vi "Initialize Generate.vi"(8 "error in (no error)":errorcluster, 10 "PCL (usec)":u32, 11 "OnCompile Variables":T12={"Name"="", "XNET Settings"={"Database"="", "Cluster"="", "Port"="", "Baud rate [Bd]"=500000, "Termination"=1, "CAN I/O Mode"=0, "FD Baud rate [Bd]"=500000, "Priority"=100, "Use Legacy"=FALSE, "FD ISO Mode"=0}, "Frames"=[], "986x Support"={"Enable"=FALSE, "RIO Device"="", "Bitfile"=path ""}, "Incoming Signal Info"={"Signal Settings Out"=[], "Signal_Valid_Values"=[], "Signal Names"=[]}, "Incoming Frames"=[]} {"Incoming Frames"."Protection Configurations"."CRC Channels"."Data Type" items=["Signed", "Unsigned", "IEEE Float"]; "Incoming Signal Info"."Signal Settings Out"."Protection Configuration"."CRC Channels"."Data Type" items=["Signed", "Unsigned", "IEEE Float"]; "XNET Settings"."FD ISO Mode" items=["ISO", "Non ISO", "ISO Legacy"]; "XNET Settings"."CAN I/O Mode" items=["CAN 2.0", "CAN FD", "CAN FD+BRS"]; "XNET Settings"."Termination" items=["Off", "On"]; "Frames"."Protection Configurations"."CRC Channels"."Data Type" items=["Signed", "Unsigned", "IEEE Float"]}) -> (0 "error out":errorcluster, 3 "RT Configuration":T1={"Name"="", "Priority"=100, "CAN Session"="", "Frame Count"=0, "Frames"=[], "FPGA Session"=0, "XNET Settings"={"Database"="", "Cluster"="", "Port"="", "Baud rate [Bd]"=0, "Termination"=0, "CAN I/O Mode"=0, "FD Baud rate [Bd]"=500000, "Priority"=100, "Use Legacy"=FALSE, "FD ISO Mode"=0}, "Incoming Frame Session"="", "Incoming Session Invalid"=FALSE, "Incoming Signal Info"={"Signal_Valid_Values"=[], "Signal Names"=[], "Signal Settings Out"=[], "Frame Receive Time Values"=[]}, "Signal Values"=[]} {"Incoming Signal Info"."Signal Settings Out"."Protection Configuration"."CRC Channels"."Data Type" items=["Signed", "Unsigned", "IEEE Float"]; "XNET Settings"."FD ISO Mode" items=["ISO", "Non ISO", "ISO Legacy"]; "XNET Settings"."CAN I/O Mode" items=["CAN 2.0", "CAN FD", "CAN FD+BRS"]; "XNET Settings"."Termination" items=["Off", "On"]; "Frames"."Protection Configurations"."CRC Channels"."Data Type" items=["Signed", "Unsigned", "IEEE Float"]})   [LabVIEW 2019, in "Protection and Counter Addon Engine.lvlib"]
uses:
  Protection and Counter Addon Engine.lvlib
  Addon Shared/Types/Exported.OnCompile.ctl
  Addon Shared/Types/XNET Settings.ctl
  SubModules/Frame-Protection-Support/Source/Shared/Types/Exported Frame Settings.ctl
  SubModules/Frame-Protection-Support/Source/Shared/Types/Exported Frame Type.ctl
  SubModules/Frame-Protection-Support/Source/Shared/Types/Exported Protection Settings.ctl
  SubModules/Frame-Protection-Support/Source/Shared/Types/Protection Type.ctl
  SubModules/Frame-Protection-Support/Source/Shared/Types/XNET Signal Configuration.ctl
  SubModules/Frame-Protection-Support/Source/Shared/Types/Exported Counter Settings.ctl
  SubModules/Frame-Protection-Support/Source/Shared/Types/Exported Event Trigger Type.ctl
  Addon Shared/Types/986x.ctl
  SubModules/Frame-Protection-Support/Source/Shared/Types/Incoming Signal Info.ctl
  SubModules/Frame-Protection-Support/Source/Shared/Types/Exported Signal Settings.ctl
  Types/RT Async Engine Settings.ctl
  SubModules/Frame-Protection-Support/Source/Engine/Types/RT Frame Settings.ctl
  SubModules/Frame-Protection-Support/Source/Engine/Types/RT Protection Configuration.ctl
  SubModules/Frame-Protection-Support/Source/Shared/Types/RT_Incoming_Signal_Info.ctl
  SubModules/Frame-Protection-Support/Source/Shared/Types/RT Exported Signal Settings.ctl
  <vilib>/xnet/xnet.llb/XNET Create Session (Frame Output Stream).vi
  SubModules/Frame-Protection-Support/Source/Shared/Protection and Counter Support Shared.lvlib
  SubModules/Frame-Protection-Support/Source/Engine/Protection and Counter Support Engine.lvlib
  <resource>/objmgr/xnet.rc
  Addon Shared/Protection and Counter Addon Shared.lvlib
  <vilib>/NI VeriStand/Custom Device Tools/Custom Device Utility Library/Custom Device Utility Library.lvlib
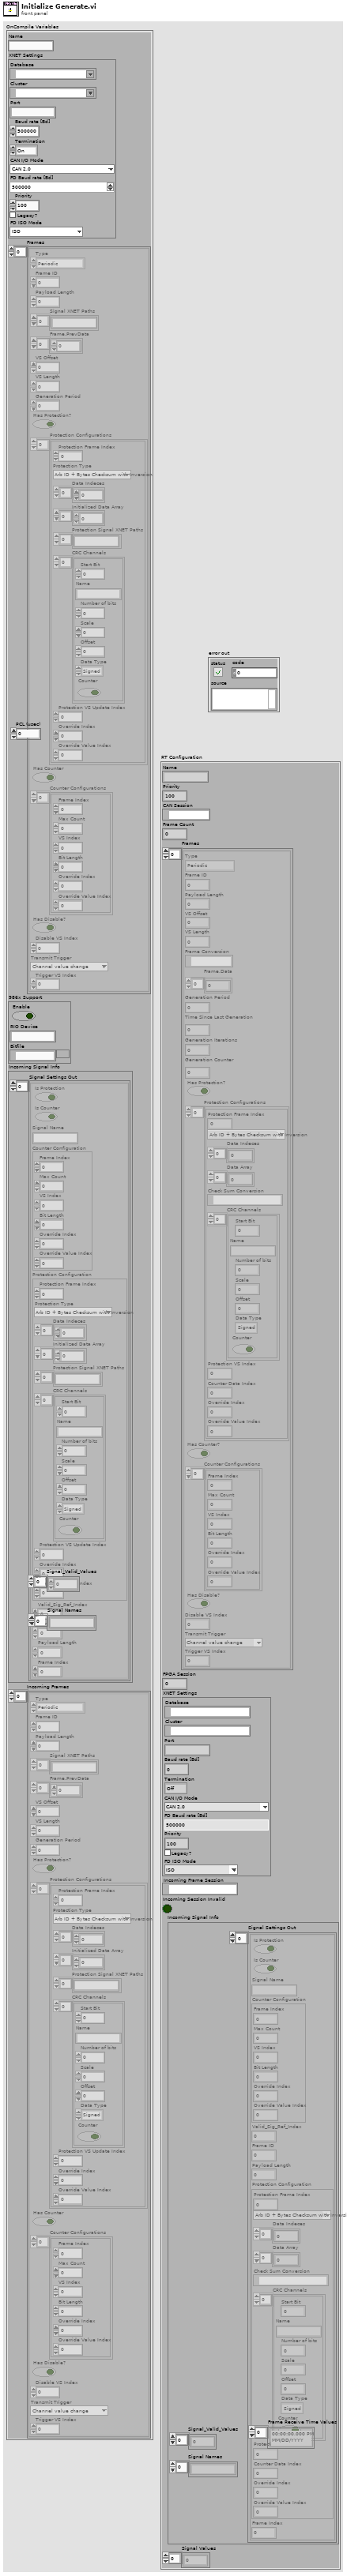
[diagram p1: front panel]
types:
  T1 = typedef "Protection and Counter Addon Engine.lvlib/RT Async Engine Settings.ctl" = cluster{"Name":string, "Priority":i32, "CAN Session":refnum<k21>, "Frame Count":i32, "Frames":T2[], "FPGA Session":u32, "XNET Settings":T9, "Incoming Frame Session":refnum<k21>, "Incoming Session Invalid":bool, "Incoming Signal Info":T10, "Signal Values":dbl[]}
  T2 = typedef "Protection and Counter Support Engine.lvlib/RT Frame Settings.ctl" = cluster{"Type":T3, "Frame ID":u32, "Payload Length":u32, "VS Offset":i32, "VS Length":i32, "Frame Conversion":refnum<k21>, "Frame.Data":dbl[], "Generation Period":u32, "Time Since Last Generation":u32, "Generation Iterations":u32, "Generation Counter":u32, "Has Protection?":bool, "Protection Configurations":T4[], "Has Counter?":bool, "Counter Configurations":T7[], "Has Disable?":bool, "Disable VS Index":i32, "Transmit Trigger":T8, "Trigger VS Index":i32}
  T3 = typedef "Protection and Counter Support Shared.lvlib/Exported Frame Type.ctl" = enum16{"Periodic", "Event", "Periodic/Event"}
  T4 = typedef "Protection and Counter Support Engine.lvlib/RT Protection Configuration.ctl" = cluster{"Protection Frame Index":i32, "Protection Type":T5, "Data Indeces":i32[], "Data Array":dbl[], "Check Sum Conversion":refnum<k21>, "CRC Channels":T6[], "Protection VS Index":i32, "Counter Data Index":i32, "Override Index":i32, "Override Value Index":i32}
  T5 = typedef "Protection and Counter Support Shared.lvlib/Protection Type.ctl" = enum16{"Arb ID + Bytes Checksum with Inversion", "Arb ID + Bytes CRC with Inversion", "Reversed Raw Signal Checksum with Inversion", "Concatenated Two's Compliment"}
  T6 = typedef "Protection and Counter Support Shared.lvlib/XNET Signal Configuration.ctl" = cluster{"Start Bit":i32, "Name":string, "Number of bits":i32, "Scale":dbl, "Offset":dbl, "Data Type":u32, "Counter":bool}
  T7 = typedef "Protection and Counter Support Shared.lvlib/Exported Counter Settings.ctl" = cluster{"Frame Index":i32, "Max Count":dbl, "VS Index":i32, "Bit Length":i64, "Override Index":i32, "Override Value Index":i32}
  T8 = typedef "Protection and Counter Support Shared.lvlib/Exported Event Trigger Type.ctl" = enum16{"Channel value change", "Trigger channel (not zero)", "Channel value change or trigger channel (not zero)", "Trigger channel (any value change)", "Channel value change or trigger channel (any value change)"}
  T9 = typedef "Protection and Counter Addon Shared.lvlib/XNET Settings.ctl" = cluster{"Database":refnum<k21>, "Cluster":refnum<k21>, "Port":string, "Baud rate [Bd]":u64, "Termination":u32, "CAN I/O Mode":u32, "FD Baud rate [Bd]":u64, "Priority":i32, "Use Legacy":bool, "FD ISO Mode":u32}
  T10 = typedef "RT_Incoming_Signal_Info.ctl" = cluster{"Signal_Valid_Values":dbl[], "Signal Names":string[], "Signal Settings Out":T11[], "Frame Receive Time Values":timestamp[]}
  T11 = typedef "RT Exported Signal Settings.ctl" = cluster{"Is Protection":bool, "Is Counter":bool, "Signal Name":string, "Counter Configuration":T7, "Valid_Sig_Ref_Index":i32, "Frame ID":u32, "Payload Length":u32, "Protection Configuration":T4, "Frame Index":i32}
  T12 = typedef "Protection and Counter Addon Shared.lvlib/Exported.OnCompile.ctl" = cluster{"Name":string, "XNET Settings":T9, "Frames":T13[], "986x Support":T15, "Incoming Signal Info":T16, "Incoming Frames":T13[]}
  T13 = typedef "Protection and Counter Support Shared.lvlib/Exported Frame Settings.ctl" = cluster{"Type":T3, "Frame ID":u32, "Payload Length":u32, "Signal XNET Paths":string[], "Frame.PrevData":dbl[], "VS Offset":i32, "VS Length":i32, "Generation Period":u32, "Has Protection?":bool, "Protection Configurations":T14[], "Has Counter":bool, "Counter Configurations":T7[], "Has Disable?":bool, "Disable VS Index":i32, "Transmit Trigger":T8, "Trigger VS Index":i32}
  T14 = typedef "Protection and Counter Support Shared.lvlib/Exported Protection Settings.ctl" = cluster{"Protection Frame Index":i32, "Protection Type":T5, "Data Indeces":i32[], "Initialized Data Array":dbl[], "Protection Signal XNET Paths":string[], "CRC Channels":T6[], "Protection VS Update Index":i32, "Override Index":i32, "Override Value Index":i32}
  T15 = typedef "Protection and Counter Addon Shared.lvlib/986x.ctl" = cluster{"Enable":bool, "RIO Device":string, "Bitfile":path}
  T16 = typedef "Incoming Signal Info.ctl" = cluster{"Signal Settings Out":T17[], "Signal_Valid_Values":dbl[], "Signal Names":string[]}
  T17 = typedef "Exported Signal Settings.ctl" = cluster{"Is Protection":bool, "Is Counter":bool, "Signal Name":string, "Counter Configuration":T7, "Protection Configuration":T14, "Valid_Sig_Ref_Index":i32, "Frame ID":u32, "Payload Length":u32, "Frame Index":i32}
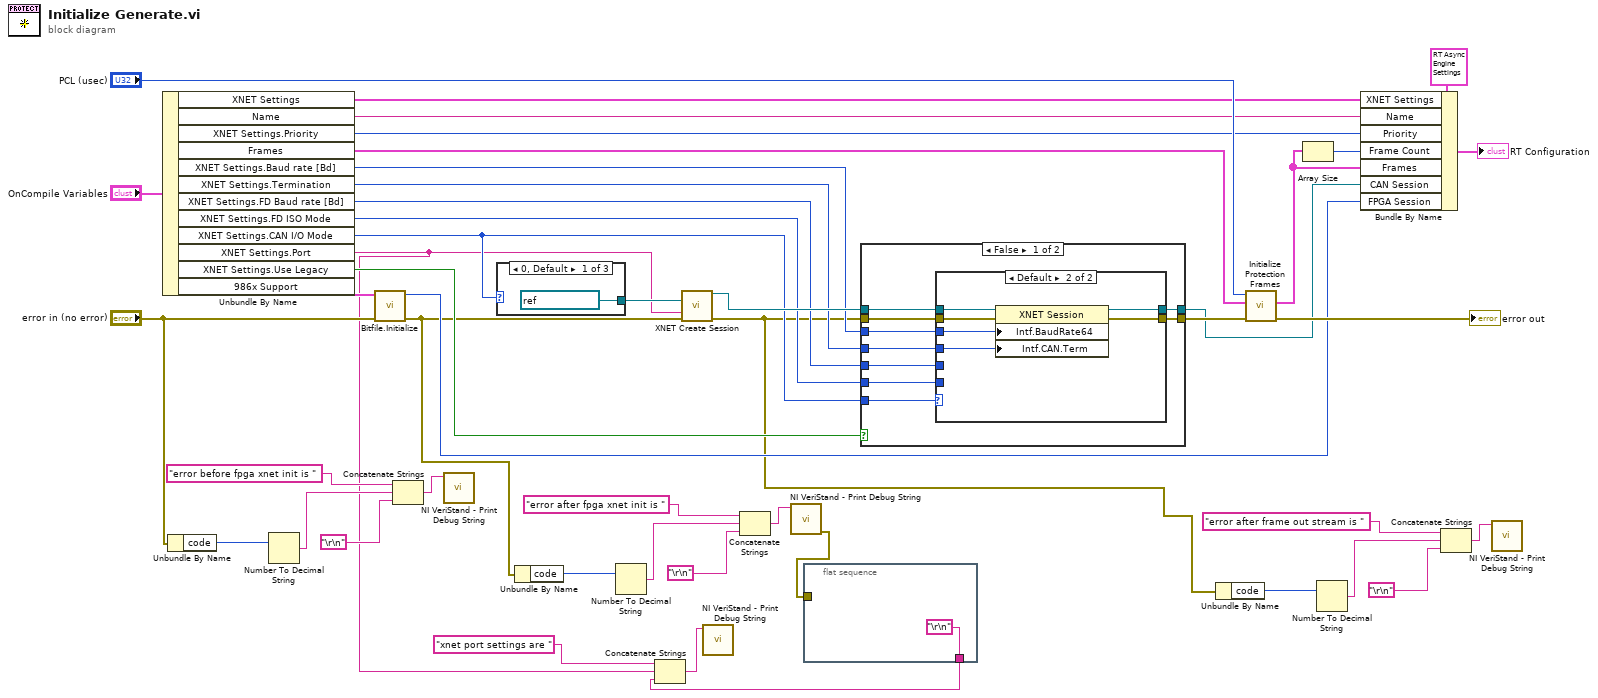
[diagram p0: block diagram]
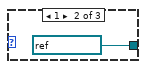
[diagram p2: hidden frame]
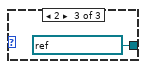
[diagram p3: hidden frame]
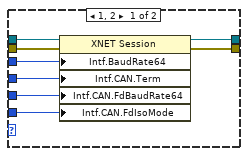
[diagram p4: hidden frame]
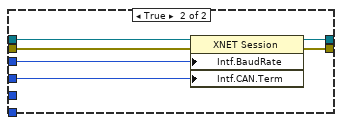
[diagram p5: hidden frame]
diagram:
  n1 = Unbundle By Name("OnCompile Variables") -> ("XNET Settings"=w27:T9, "Name"=w28:string, "XNET Settings.Priority"=w34:i32, "Frames"=w45:T13[], "XNET Settings.Baud rate [Bd]"=w37:u64, "XNET Settings.Termination"=w38:u32, "XNET Settings.FD Baud rate [Bd]"=w39:u64, "XNET Settings.FD ISO Mode"=w25:u32, "XNET Settings.CAN I/O Mode"=w24:u32, "XNET Settings.Port"=w3:string, "XNET Settings.Use Legacy"=w33:bool, "986x Support"=w32:T15)
  n2 = Unbundle By Name("error in (no error)") -> ("code"=w19:i32)
  n3 = Number To Decimal String(number=w19) -> (decimal integer string=w21:string)  [unwired: 1 in]
  n4 = call "Bitfile.Initialize.vi"("error in (no error)"="error in (no error)", "FPGA Bitfile Settings"=w32) -> ("error out"=w12:errorcluster, "FPGA Session"=w31:u32)  [unwired: 8 in]
  n5 = Concatenate Strings("error before fpga xnet init is " ("string"), w21, "\r\n") -> (w23:string)
  n6 = call <vilib>:"NI VeriStand - Print Debug String.vi"("Message"=w23) -> ()  [unwired: 10 in, 1 out]
  n7 = case shown="0, Default" w24 {
    tunnel: [refnum<k21> ":memory:" ("cluster (:memory:)") refnum<k21> ":can_fd:" ("cluster (:memory:)") refnum<k21> ":can_fd_brs:" ("cluster (:memory:)")] -> w26
    frame 0, Default {
    }
    frame 1 {
    }
    frame 2 {
    }
  }
  n8 = Unbundle By Name(w12) -> ("code"=w13:i32)
  n9 = Number To Decimal String(number=w13) -> (decimal integer string=w15:string)  [unwired: 1 in]
  n10 = Concatenate Strings("xnet port settings are " ("string"), w3, w1) -> (w5:string)
  n11 = call-poly <vilib>:"XNET Create Session.vi"("cluster (:memory:)"=w26, "interface"=w3, "error in (no error)"=w12) -> ("session out"=w41:refnum<k21>, "error out"=w6:errorcluster)  [unwired: 11 in]
  n12 = call <vilib>:"NI VeriStand - Print Debug String.vi"("Message"=w5) -> ()  [unwired: 10 in, 1 out]
  n13 = Concatenate Strings("error after fpga xnet init is " ("string"), w15, "\r\n") -> (w17:string)
  n14 = call <vilib>:"NI VeriStand - Print Debug String.vi"("Message"=w17) -> ("error out"=w2:errorcluster)  [unwired: 10 in]
  n15 = flat-sequence {
    tunnel: w2 -> [_]
    tunnel: ["\r\n"] -> w1
    frame #0 {
    }
  }
  n16 = case shown="False" w33 {
    tunnel: w6 -> [w59 w79]
    tunnel: w41 -> [w58 w78]
    tunnel: [w57 w77] -> w40
    tunnel: w39 -> [w56 _]
    tunnel: w24 -> [w52 _]
    tunnel: w38 -> [w55 w74]
    tunnel: w37 -> [w54 w75]
    tunnel: [w53 w76] -> w29
    tunnel: w25 -> [w51 _]
    frame False {
      n17 = case shown="Default" w52 {
        tunnel: w59 -> [w67 w73]
        tunnel: w58 -> [w66 w72]
        tunnel: [w65 w71] -> w57
        tunnel: w56 -> [w64 _]
        tunnel: w55 -> [w63 w70]
        tunnel: w54 -> [w62 w69]
        tunnel: [w61 w68] -> w53
        tunnel: w51 -> [w60 _]
        frame 1, 2 {
          n18 = property class="XNET Session"(reference=w66, error in=w67, "Intf.BaudRate64"=w62, "Intf.CAN.Term"=w63, "Intf.CAN.FdBaudRate64"=w64, "Intf.CAN.FdIsoMode"=w60) -> (reference out=w61:refnum<k21>, error out=w65:errorcluster)
        }
        frame Default {
          n19 = property class="XNET Session"(reference=w72, error in=w73, "Intf.BaudRate64"=w69, "Intf.CAN.Term"=w70) -> (reference out=w68:refnum<k21>, error out=w71:errorcluster)
        }
      }
    }
    frame True {
      n20 = property class="XNET Session"(reference=w78, error in=w79, "Intf.BaudRate"=w75, "Intf.CAN.Term"=w74) -> (reference out=w76:refnum<k21>, error out=w77:errorcluster)
    }
  }
  n21 = Unbundle By Name(w6) -> ("code"=w7:i32)
  n22 = call "Initialize Protection Frames.vi"("error in (no error)"=w40, "Frames"=w45, "PCL (usec)"="PCL (usec)") -> ("error out"=→"error out":errorcluster, "RT Frames"=w30:T2[])  [unwired: 7 in]
  n23 = Array Size(array=w30) -> (size(s)=w35:i32)
  n24 = Number To Decimal String(number=w7) -> (decimal integer string=w9:string)  [unwired: 1 in]
  n25 = Bundle By Name(cluster=T1 {"Name"="", "Priority"=100, "CAN Session"="", "Frame Count"=0, "Frames"=[], "FPGA Session"=0, "XNET Settings"={"Database"="", "Cluster"="", "Port"="", "Baud rate [Bd]"=0, "Termination"=0, "CAN I/O Mode"=0, "FD Baud rate [Bd]"=500000, "Priority"=100, "Use Legacy"=FALSE, "FD ISO Mode"=0}, "Incoming Frame Session"="", "Incoming Session Invalid"=FALSE, "Incoming Signal Info"={"Signal_Valid_Values"=[], "Signal Names"=[], "Signal Settings Out"=[], "Frame Receive Time Values"=[]}, "Signal Values"=[]} ("RT Configuration"), "XNET Settings"=w27, "Name"=w28, "Priority"=w34, "Frame Count"=w35, "Frames"=w30, "CAN Session"=w29, "FPGA Session"=w31) -> (→"RT Configuration":T1)
  n26 = Concatenate Strings("error after frame out stream is " ("string"), w9, "\r\n") -> (w11:string)
  n27 = call <vilib>:"NI VeriStand - Print Debug String.vi"("Message"=w11) -> ()  [unwired: 10 in, 1 out]
